vi "Plotmatrix Format Page.vi"() -> ()   [LabVIEW 2020, in "XY Plot Matrix.lvclass"]
uses:
  <vilib>/Math Plots/2D Math Plots/XY Plot Matrix/XY Plot Matrix/XY Plot Matrix.lvclass
  <vilib>/Math Plots/2D Math Plots/2D Plot/Action String/XYPlotMatrix Ctrl Act Queue.ctl
  <vilib>/Math Plots/2D Math Plots/2D Plot/Action String/XYPlotMatrix Ctrl Act Cluster.ctl
  <vilib>/Math Plots/2D Math Plots/2D Plot/Action String/2DMathPlot State Class.ctl
  <vilib>/Math Plots/2D Math Plots/2D Plot/2D Plot/Typedef/Dialog State.ctl
  <vilib>/Math Plots/2D Math Plots/2D Plot/2D Plot/Typedef/Temp Graph State.ctl
  <vilib>/Math Plots/2D Math Plots/2D Plot/2D Plot/Typedef/Temp Graph Property Action.ctl
  <vilib>/Math Plots/2D Math Plots/2D Plot/2D Plot/2D Plot.lvclass
panel:
  in  "Axis":string[](array[string])=["(X-Axis)", "(Y-Axis)"]
  in  "Current Scale":u16(ring)
  in  "Control Ref Queue":T1
  out "Format String Out":string[](array[string])
  in  "Format String In":string[](array[string])
  out "Advanced Tab":enum32{"Standard", "Advanced"}(tab)
  in  "Type":i32(listbox)
  out "Time/Date Tab":enum32{"numeric", "time"}(tab) caption="Tab Control 3"
  in  "HLP_just/pad":i32(ring) items=["Pad with spaces on left", "Pad with spaces on right", "Pad with zeros on left"]
  in  "HLP_Minimum field width":i32 caption="Minimum field width" min=0
  in  "Digits":i32 min=0
  in  "Precision Type":u16(ring) items=["Digits of precision", "Significant digits"]
  in  "HLP_exponent":bool caption="Exponent in multiples of 3"
  in  "HLP_trailing zeros":bool caption="Hide trailing zeros"
  in  "HLP_UseMinWidth":bool caption="Use minimum field width"
  in  "HLP_Date Type":u16(ring)=1 caption="Date Type" items=["Custom date format", "System date format", "Date unused"]
  in  "HLP_MDY 2-new":T2(radio)
  in  "HLP_year-new":T2(radio)
  in  "HLP_Time Type":u16(ring)=1 caption="Time Type" items=["Custom time format", "System time format", "Time unused"]
  in  "HLP_Digits":i32 caption="Digits" min=0
  in  "HLP_Hour Type-new":enum32{"Radio Selection 1", "Radio Selection 2"}(radio)
  in  "HLP_HMS-new":enum32{"Radio Selection 1", "Radio Selection 2"}(radio)
  in  "HLP_Format Code List Type":u16(ring) items=["Numeric format codes", "Relative time format codes", "Absolute time format codes"]
  in  "ODF_Format String":string caption="Format string"
  in  "HLP_percent codes":i32(listbox) caption="Numeric Format Codes"
  in  "HLP_insert format code":bool caption="Insert into Format String"
  out "HLP_Valid Fmt String":bool=TRUE caption="Valid"
  in  "HLP_Revert":bool caption="Revert"
  in  "HLP_AdvancedFmt2":enum32{"Default mode", "Advanced mode"}(radio)
  in  "Event Registration":refnum<event-registration>
  in  "Item Names":string[][][](array[string])=[[["Floating point notation", "%f"], ["Scientific notation", "%e"], ["Engineering notation", "%^e"], ["Automatic notation", "%#_g"], ["SI notation", "%p"], ["Decimal", "%d"], ["Unsigned decimal", "%u"], ["Hexadecimal", "%x"], ["Octal", "%o"], ["Binary", "%b"], ["A single percent character", "%%"], ["", ""], ["", ""], ["", ""], ["", ""], ["", ""], ["", ""], ["", ""], ["", ""], ["", ""], ["", ""], ["", ""], ["", ""]], [["Absolute time container", "%< >T"], ["Abbreviated weekday name", "%a"], ["Weekday name", "%A"], ["Abbreviated month name", "%b"], ["Month name", "%B"], ["Default date and time", "%c"], ["Day of month (01-31)", "%d"], ["Hour (24-hour clock) (00-23)", "%H"], ["Hour (12-hour clock) (01-12)", "%I"], ["Day of year (001-366)", "%j"], ["Month number (01-12)", "%m"], ["Minute (00-59)", "%M"], ["AM or PM flag", "%p"], ["Seconds (00-59)", "%S"], ["Fractional seconds with <digit>\nprecision", "%<digit> u"], ["Week number (00-53) with\nSunday as the first day of week 1", "%U"], ["Weekday number (0-6)", "%w"], ["Week number (00-53) with\nMonday as the first day of week 1", "%W"], ["Locale date", "%x"], ["Locale time", "%X"], ["Year within century (00-99)", "%y"], ["Year including century", "%Y"], ["Time zone", "%Z"]], [["Relative time container", "%< >t"], ["Weeks", "%W"], ["Days", "%D"], ["Hours", "%H"], ["Minutes", "%M"], ["Seconds", "%S"], ["Fractional seconds with <digit>\nprecision", "%<digit>u"], ["A single percent character", "%%"], ["", ""], ["", ""], ["", ""], ["", ""], ["", ""], ["", ""], ["", ""], ["", ""], ["", ""], ["", ""], ["", ""], ["", ""], ["", ""], ["", ""], ["", ""]]]
  in  "Caption Texts":string[](array[string])=["Numeric Format Codes", "Absolute Time Format Codes\n(must be within %< >T)", "Relative Time Format Codes\n(must be within %< >t)"]
  out "Format test string":string
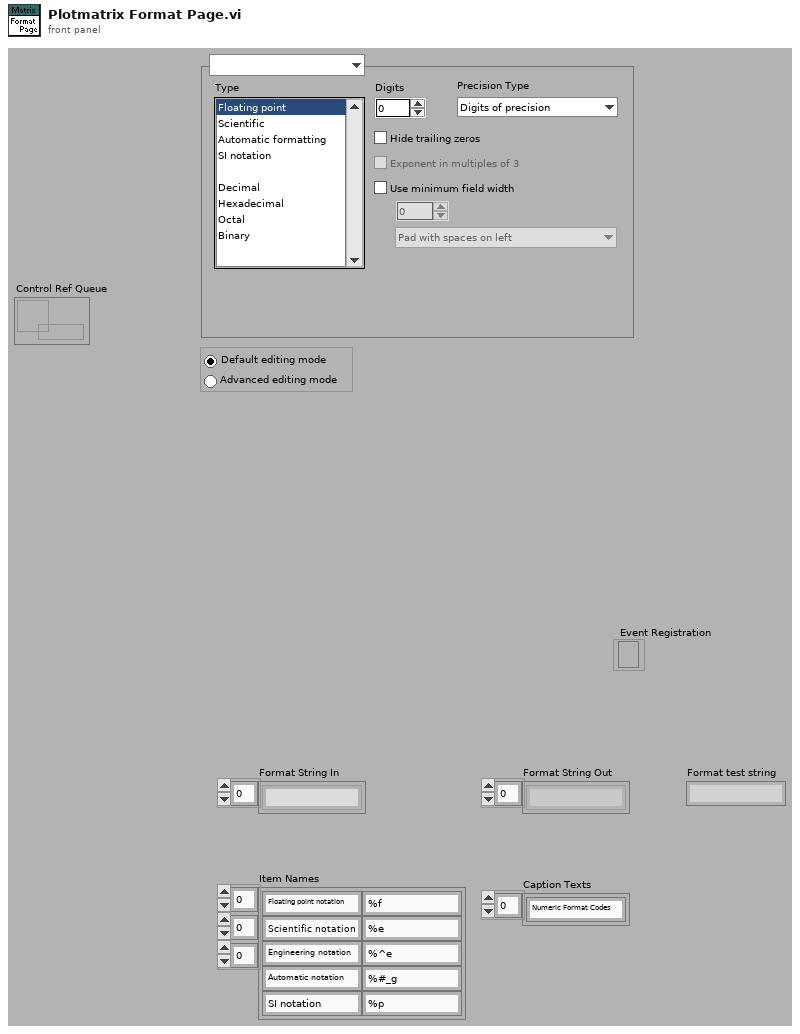
[diagram p1: front panel]
types:
  T1 = typedef "XYPlotMatrix Ctrl Act Queue.ctl" = refnum<queue>
  T2 = enum32{"Radio Selection 1", "Radio Selection 2", "Radio Selection 3"}
  T3 = typedef "2D Plot.lvclass/Dialog State.ctl" = enum16{"Initialize", "Read Property", "Write Property", "Idle", "Exit"}
  T4 = typedef "2D Plot.lvclass/Temp Graph State.ctl" = enum16{"Create", "Update Graph", "Update Property Only", "Get Plot Name", "Get Axis Name", "Destory"}
  T5 = typedef "2D Plot.lvclass/Temp Graph Property Action.ctl" = enum16{"Appearance Property", "Format Property", "Plots Property", "Scales Property"}
  T6 = enum16{"number", "absolute time", "relative time"}
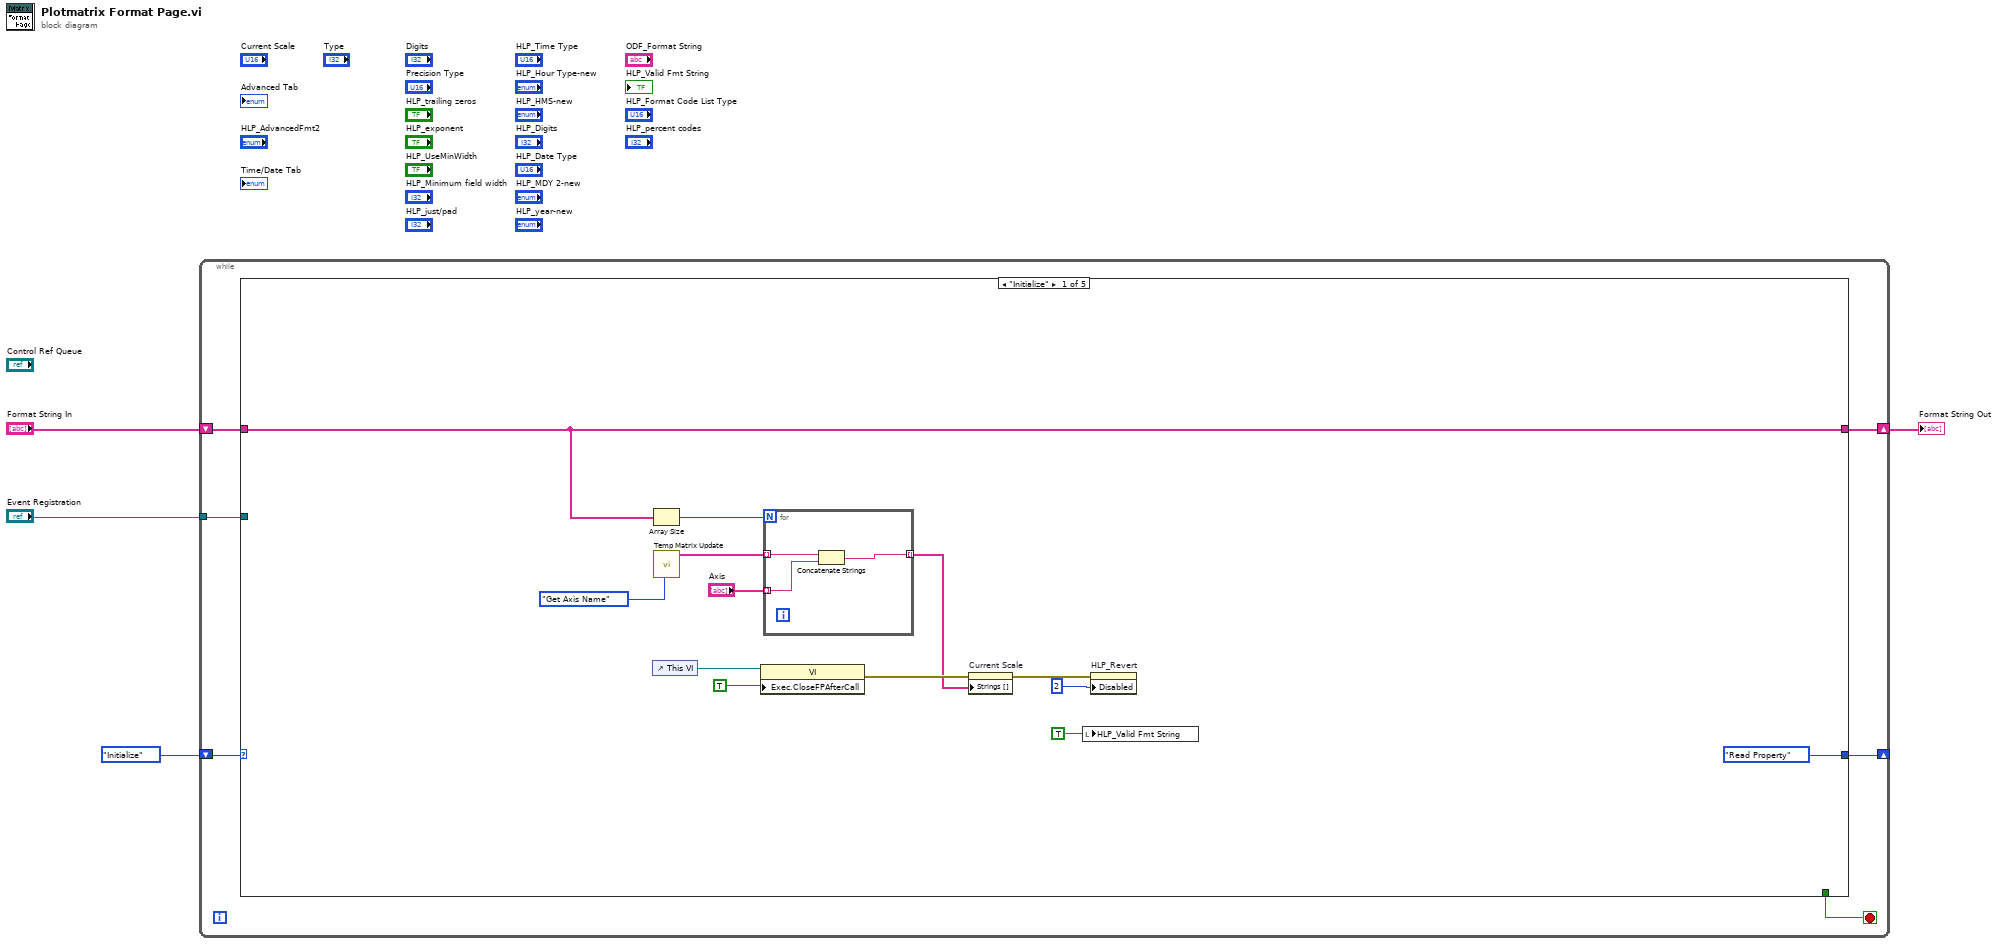
[diagram p0: block diagram]
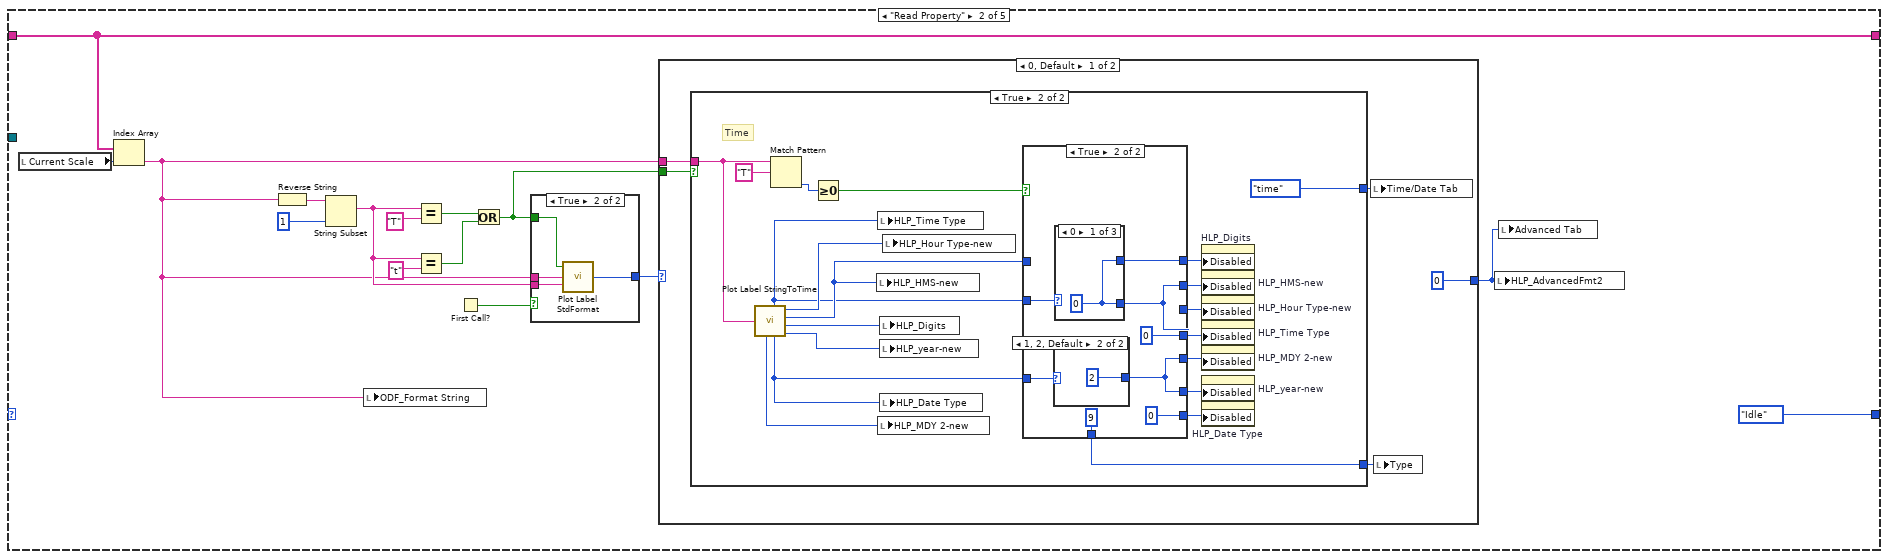
[diagram p2: hidden frame]
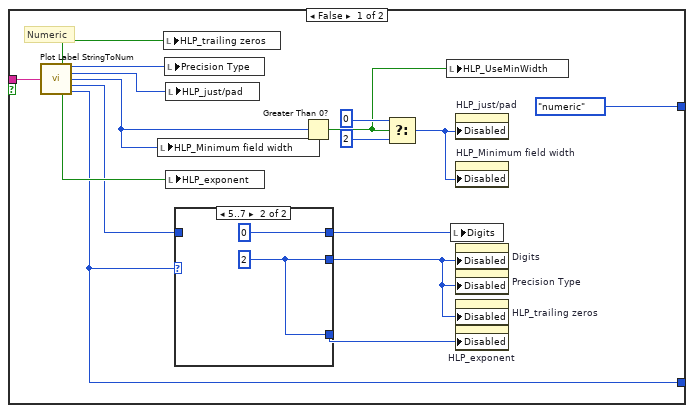
[diagram p3: hidden frame]
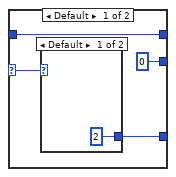
[diagram p4: hidden frame]
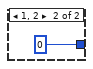
[diagram p5: hidden frame]
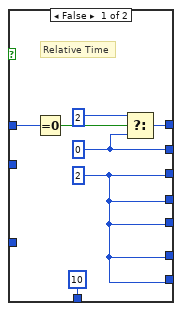
[diagram p6: hidden frame]
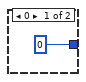
[diagram p7: hidden frame]
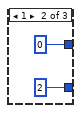
[diagram p8: hidden frame]
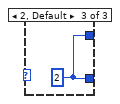
[diagram p9: hidden frame]
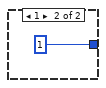
[diagram p10: hidden frame]
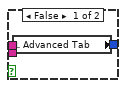
[diagram p11: hidden frame]
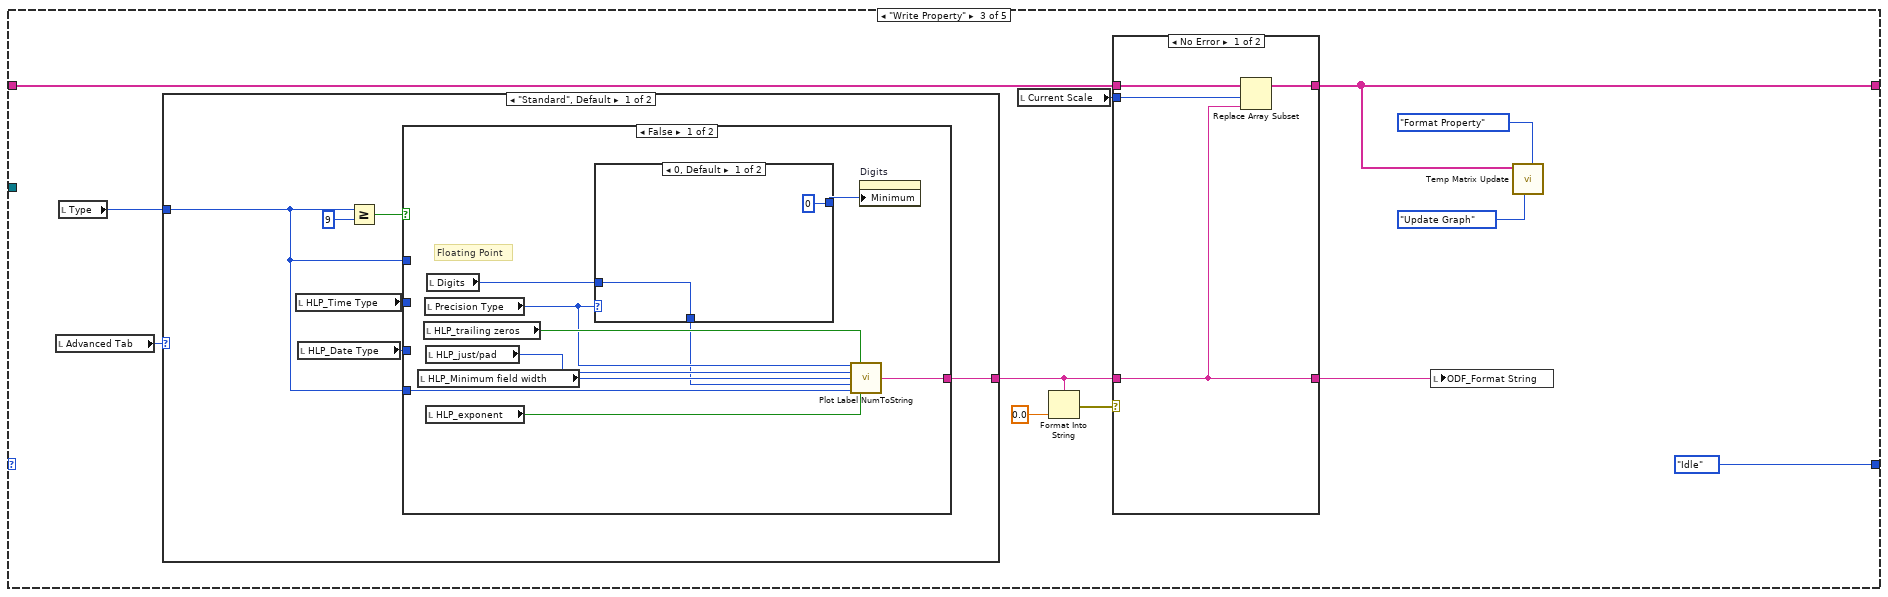
[diagram p12: hidden frame]
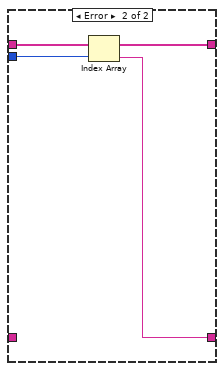
[diagram p13: hidden frame]
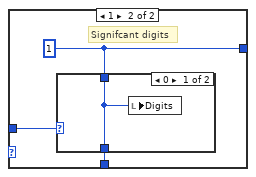
[diagram p14: hidden frame]
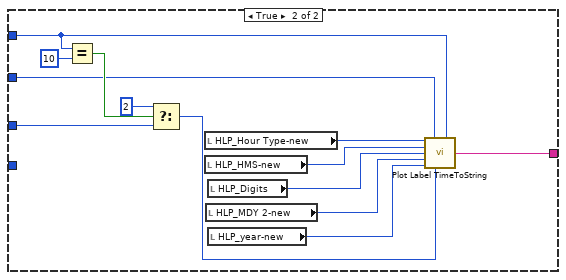
[diagram p16: hidden frame]
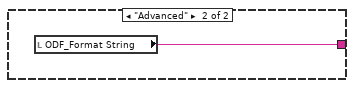
[diagram p17: hidden frame]
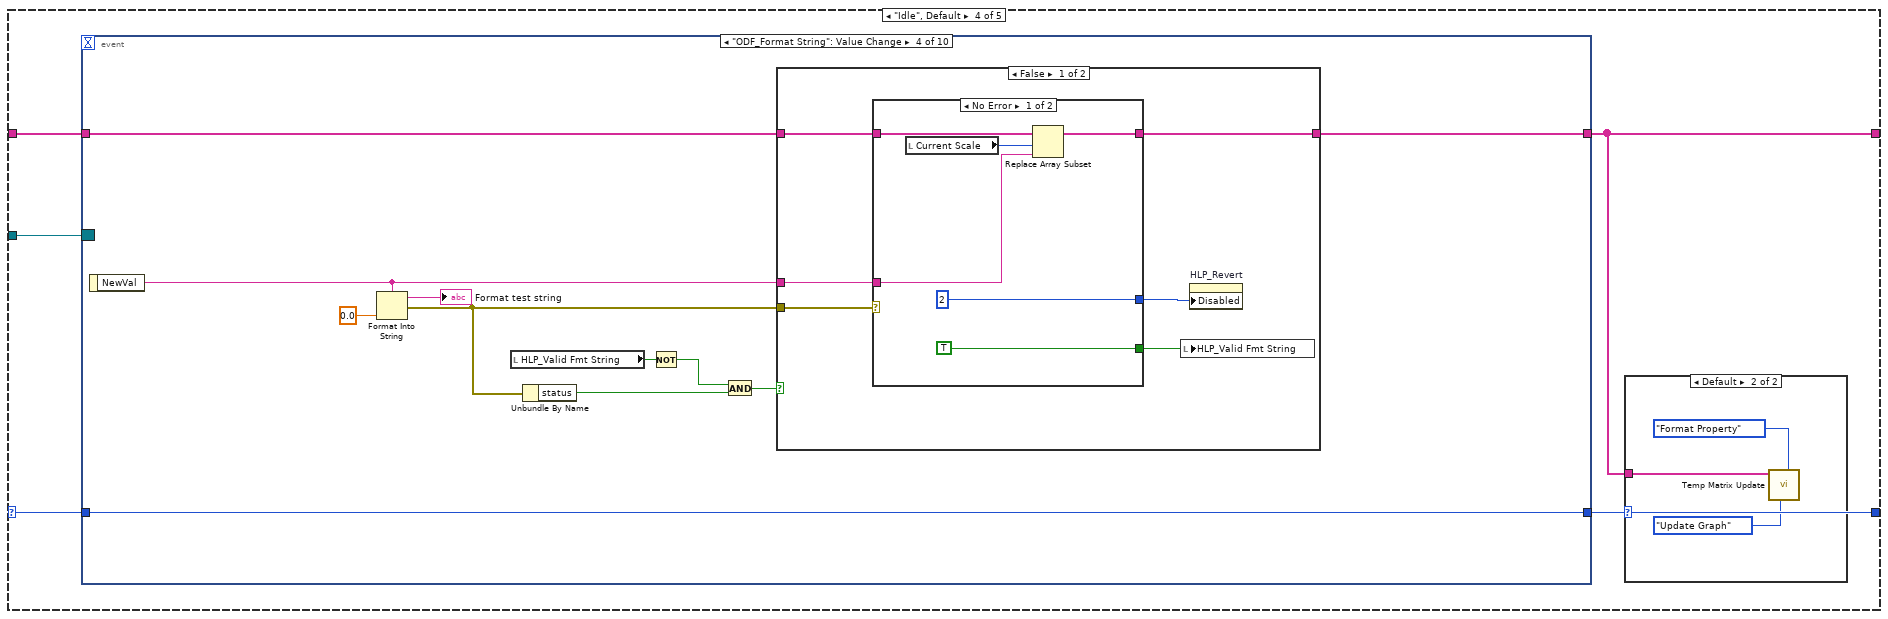
[diagram p18: hidden frame]
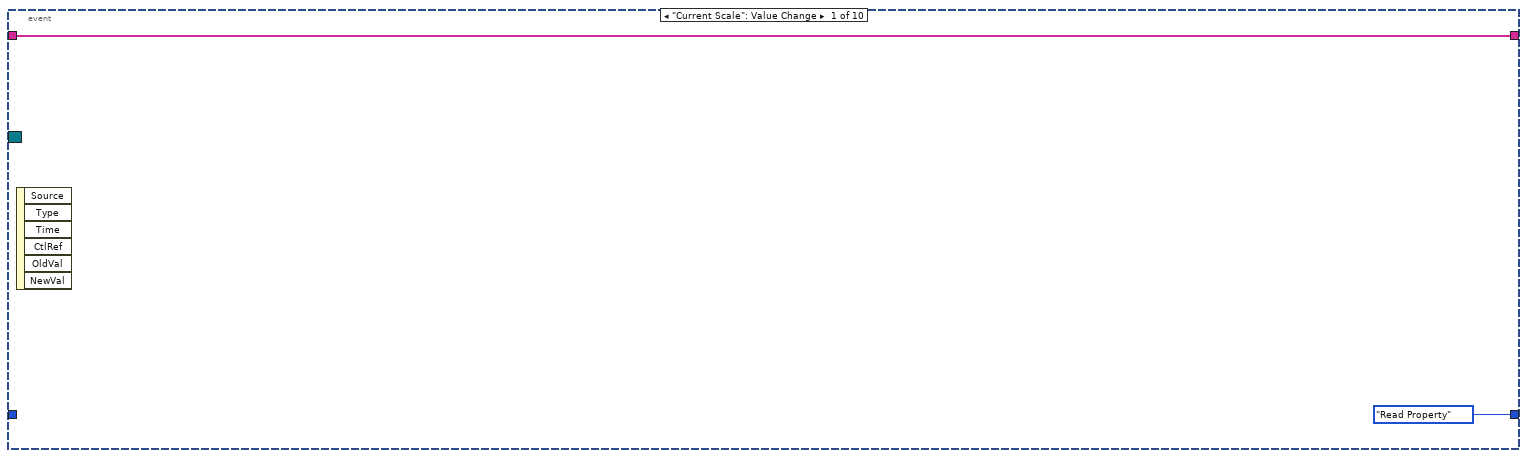
[diagram p20: hidden frame]
diagram:
  n1 = while {
    shift-right: [w5] -> w2
    shift-left: "Format String In" -> [w10]
    shift-right: [w6] -> _
    shift-left: Dialog_State."Initialize" ("Enum") -> [w7]
    tunnel: "Event Registration" -> [w8]
    stop <- w9 stop-if-true
    n2 = case shown="\"Initialize\"" w7 {
      selector: w7 -> [_ _ _ w176 _]
      tunnel: w10 -> [w13 w40 w121 w178 w401]
      tunnel: [w13 w40 w118 w175 w401] -> w5
      tunnel: [Dialog_State."Read Property" ("Enum") Dialog_State."Idle" ("Enum") Dialog_State."Idle" ("Enum") w174 Dialog_State."Exit" ("Enum")] -> w6
      tunnel: [_ _ _ _ TRUE] -> w9
      tunnel: w8 -> [_ _ _ w177 _]
      frame "Initialize" {
        n3 = control-ref of="This VI"() -> (w23:refnum<vi>)
        n4 = Array Size(array=w13) -> (size(s)=w12:i32)
        n5 = call <vilib>:"Temp Matrix Update.vi"("State"=Temp_Graph_State."Get Axis Name") -> ("Item Strings"=w15:string[])  [unwired: 4 in, 6 out]
        n6 = property class="VI"(reference=w23, "Exec.CloseFPAfterCall"=TRUE ("Execution:Close After Call")) -> (error out=w18:errorcluster)  [unwired: 1 in, 1 out]
        n7 = for {
          N: w12 -> [_]
          tunnel: w15 -> [w26] mode=indexing
          tunnel: [w24] -> w14 mode=indexing
          tunnel: "Axis" -> [w25] mode=indexing
          n8 = Concatenate Strings(w26, w25) -> (w24:string)
        }
        n9 = property on="Current Scale" class="Ring (strict)"(error in=w18, "Strings []"=w14) -> (error out=w17:errorcluster)  [unwired: 1 in, 1 out]
        n10 = local write "HLP_Valid Fmt String"(TRUE ("HLP_Valid Fmt String")) -> ()
        n11 = property on="HLP_Revert" class="Bool"(error in=w17, "Disabled"=u8 2) -> ()  [unwired: 1 in, 2 out]
      }
      frame "Read Property" {
        n12 = local read "Current Scale"() -> (w41:u16)
        n13 = Index Array(array=w40, index=w41) -> (element=w30:string)
        n14 = Reverse String(1:w30) -> (0:w35:string)
        n15 = String Subset(string=w35, length (rest)=1 ("length (rest)")) -> (substring=w39:string)  [unwired: 1 out]
        n16 = local write "ODF_Format String"(w30) -> ()
        n17 = Equal?(x=w39, y="T") -> (x = y?=w37:bool)
        n18 = Equal?(x=w39, y="t") -> (x = y?=w38:bool)
        n19 = First Call?() -> (First Call?: T/F=w32:bool)
        n20 = Or(x=w37, y=w38) -> (x .or. y?=w29:bool)
        n21 = case shown="True" w32 {
          tunnel: w39 -> [_ w115]
          tunnel: w29 -> [_ w117]
          tunnel: w30 -> [_ w116]
          tunnel: [w113 w114] -> w31
          frame False {
            n22 = local read "Advanced Tab"() -> (w113:enum32{"Standard", "Advanced"})
          }
          frame True {
            n23 = call <vilib>:"Plot Label StdFormat.vi"("Time Type"=w115, "Format String"=w116, "Type (false = numeric)"=w117) -> ("Custom"=w114:i32)
          }
        }
        n24 = case shown="0, Default" w31 {
          tunnel: w30 -> [w46 _]
          tunnel: w29 -> [w45 _]
          tunnel: [0 1] -> w28
          frame 0, Default {
            n25 = case shown="True" w45 {
              tunnel: w46 -> [w62 w88]
              tunnel: [w55 w79] -> w44
              tunnel: [enum32{"numeric", "time"}."numeric" ("Time/Date Tab") enum32{"numeric", "time"}."time" ("Time/Date Tab")] -> w43
              frame False {
                # "Numeric"
                n26 = call <vilib>:"Plot Label StringToNum.vi"("Format String"=w62) -> ("Hide trailing zeros"=w61:bool, "Digit Type"=w59:i32, "just/pad"=w58:i32, "Minimum Field Width"=w50:i32, "Digits of Precision"=w57:i32, "exponent"=w60:bool, "Numeric Format"=w55:i32)  [unwired: 8 out]
                n27 = local write "HLP_Minimum field width"(w50) -> ()
                n28 = local write "HLP_trailing zeros"(w61) -> ()
                n29 = local write "Precision Type"(w59) -> ()
                n30 = local write "HLP_just/pad"(w58) -> ()
                n31 = local write "HLP_exponent"(w60) -> ()
                n32 = case shown="5..7" w55 {
                  selector: w55 -> [w64 _]
                  tunnel: [u8 0 w69] -> w54
                  tunnel: w57 -> [w65 _]
                  tunnel: [w65 0 ("Digits of Precision")] -> w56
                  tunnel: [w63 w69] -> w53
                  frame Default {
                    n33 = case shown="Default" w64 {
                      tunnel: [u8 2 u8 0] -> w63
                      frame Default {
                      }
                      frame 1, 2 {
                      }
                    }
                  }
                  frame 5..7 {
                    w69 = u8 2
                  }
                }
                n34 = Greater Than 0?(x=w50) -> (x > 0?=w49:bool)
                n35 = Select(t=u8 0, s=w49, f=u8 2) -> (s? t:f=w48:u8)
                n36 = local write "HLP_UseMinWidth"(w49) -> ()
                n37 = local write "Digits"(w56) -> ()
                n38 = property on="HLP_just/pad" class="Ring (strict)"("Disabled"=w48) -> ()  [unwired: 2 in, 2 out]
                n39 = property on="HLP_Minimum field width" class="DigNum (strict)"("Disabled"=w48) -> ()  [unwired: 2 in, 2 out]
                n40 = property on="Digits" class="DigNum (strict)"("Disabled"=w54) -> ()  [unwired: 2 in, 2 out]
                n41 = property on="Precision Type" class="Ring (strict)"("Disabled"=w54) -> ()  [unwired: 2 in, 2 out]
                n42 = property on="HLP_trailing zeros" class="Bool (strict)"("Disabled"=w54) -> ()  [unwired: 2 in, 2 out]
                n43 = property on="HLP_exponent" class="Bool (strict)"("Disabled"=w53) -> ()  [unwired: 2 in, 2 out]
              }
              frame True {
                # "Time"
                n44 = call <vilib>:"Plot Label StringToTime.vi"("Time & Date Format String"=w88) -> ("MDY"=w86:i16, "Time Format"=w82:i16, "AM/PM"=w87:i16, "included seconds"=w83:i16, "Date Format"=w81:i16, "seconds precision"=w84:i16, "Year Format"=w85:i16)  [unwired: 3 out]
                n45 = Match Pattern(string=w88, regular expression="T") -> (offset past match=w90:i32)  [unwired: 4 out]
                n46 = Greater Or Equal To 0?(x=w90) -> (x >= 0?=w80:bool)
                n47 = local write "HLP_HMS-new"(w83) -> ()
                n48 = local write "HLP_Time Type"(w82) -> ()
                n49 = local write "HLP_MDY 2-new"(w86) -> ()
                n50 = local write "HLP_Digits"(w84) -> ()
                n51 = local write "HLP_year-new"(w85) -> ()
                n52 = local write "HLP_Date Type"(w81) -> ()
                n53 = local write "HLP_Hour Type-new"(w87) -> ()
                n54 = case shown="True" w80 {
                  tunnel: [w92 w105] -> w76
                  tunnel: [w97 w105] -> w75
                  tunnel: [w91 w98] -> w77
                  tunnel: [w97 0] -> w74
                  tunnel: [w97 0] -> w71
                  tunnel: [w97 w102] -> w72
                  tunnel: [w97 w102] -> w73
                  tunnel: w82 -> [_ w101]
                  tunnel: w81 -> [_ w100]
                  tunnel: [10 9] -> w79
                  tunnel: w83 -> [w93 _]
                  frame False {
                    w92 = 0
                    w97 = 2
                    # "Relative Time"
                    n55 = Equal To 0?(x=w93) -> (x = 0?=w94:bool)
                    n56 = Select(t=2, s=w94, f=w92) -> (s? t:f=w91:i32)
                  }
                  frame True {
                    n57 = case shown="1, 2, Default" w100 {
                      tunnel: [0 2] -> w102
                      frame 0 {
                      }
                      frame 1, 2, Default {
                      }
                    }
                    n58 = case shown="0" w101 {
                      tunnel: [w108 2 w111] -> w105
                      tunnel: [w108 0 w111] -> w98
                      frame 0 {
                        w108 = 0
                      }
                      frame 1 {
                      }
                      frame 2, Default {
                        w111 = 2
                      }
                    }
                  }
                }
                n59 = property on="HLP_Digits" class="DigNum (strict)"("Disabled"=w77) -> ()  [unwired: 2 in, 2 out]
                n60 = property on="HLP_HMS-new" class="RadioBtnsControl (strict)"("Disabled"=w76) -> ()  [unwired: 2 in, 2 out]
                n61 = property on="HLP_Hour Type-new" class="RadioBtnsControl (strict)"("Disabled"=w75) -> ()  [unwired: 2 in, 2 out]
                n62 = property on="HLP_Time Type" class="Ring (strict)"("Disabled"=w74) -> ()  [unwired: 2 in, 2 out]
                n63 = property on="HLP_MDY 2-new" class="RadioBtnsControl (strict)"("Disabled"=w73) -> ()  [unwired: 2 in, 2 out]
                n64 = property on="HLP_year-new" class="RadioBtnsControl (strict)"("Disabled"=w72) -> ()  [unwired: 2 in, 2 out]
                n65 = property on="HLP_Date Type" class="Ring (strict)"("Disabled"=w71) -> ()  [unwired: 2 in, 2 out]
              }
            }
            n66 = local write "Time/Date Tab"(w43) -> ()
            n67 = local write "Type"(w44) -> ()
          }
          frame 1 {
          }
        }
        n68 = local write "HLP_AdvancedFmt2"(w28) -> ()
        n69 = local write "Advanced Tab"(w28) -> ()
      }
      frame "Write Property" {
        n70 = local read "Advanced Tab"() -> (w129:enum32{"Standard", "Advanced"})
        n71 = local read "Type"() -> (w128:i32)
        n72 = case shown="\"Standard\", Default" w129 {
          tunnel: w128 -> [w140 _]
          tunnel: [w137 w173] -> w125
          frame "Standard", Default {
            n73 = local read "HLP_Time Type"() -> (w139:u16)
            n74 = local read "HLP_Date Type"() -> (w138:u16)
            n75 = Greater Or Equal?(x=w140, y=9) -> (x >= y?=w141:bool)
            n76 = case shown="False" w141 {
              tunnel: w140 -> [_ w167]
              tunnel: w140 -> [w151 _]
              tunnel: w139 -> [_ w168]
              tunnel: w138 -> [_ w169]
              tunnel: [w152 w160] -> w137
              frame False {
                # "Floating Point"
                n77 = local read "HLP_Minimum field width"() -> (w149:i32)
                n78 = local read "HLP_trailing zeros"() -> (w148:bool)
                n79 = local read "Precision Type"() -> (w146:u16)
                n80 = local read "HLP_just/pad"() -> (w147:i32)
                n81 = local read "HLP_exponent"() -> (w150:bool)
                n82 = local read "Digits"() -> (w145:i32)
                n83 = case shown="0, Default" w146 {
                  tunnel: w145 -> [w153 w157]
                  tunnel: [0 ("Data Range:Minimum") w156] -> w144
                  tunnel: [w153 w155] -> w143
                  frame 0, Default {
                  }
                  frame 1 {
                    w156 = 1 ("Data Range:Minimum")
                    # "Signifcant digits"
                    n84 = case shown="0" w157 {
                      selector: w157 -> [_ w159]
                      tunnel: w156 -> [w158 _]
                      tunnel: [w158 w159] -> w155
                      frame 0 {
                        n85 = local write "Digits"(w158) -> ()
                      }
                      frame 1, Default {
                      }
                    }
                  }
                }
                n86 = call <vilib>:"Plot Label NumToString.vi"("Digit Type"=w146, "Hide trailing zeros"=w148, "just/pad"=w147, "Minimum Field Width"=w149, "Digits of Precision"=w143, "Numeric Format"=w151, "exponent"=w150) -> ("Format String"=w152:string)  [unwired: 8 out]
                n87 = property on="Digits" class="DigNum (strict)"("Minimum"=w144) -> ()  [unwired: 2 in, 2 out]
              }
              frame True {
                n88 = Equal?(x=w167, y=10) -> (x = y?=w170:bool)
                n89 = Select(t=u16 2, s=w170, f=w169) -> (s? t:f=w161:u16)
                n90 = local read "HLP_Hour Type-new"() -> (w166:enum32{"Radio Selection 1", "Radio Selection 2"})
                n91 = local read "HLP_HMS-new"() -> (w165:enum32{"Radio Selection 1", "Radio Selection 2"})
                n92 = local read "HLP_MDY 2-new"() -> (w163:T2)
                n93 = local read "HLP_Digits"() -> (w164:i32)
                n94 = local read "HLP_year-new"() -> (w162:T2)
                n95 = call <vilib>:"Plot Label TimeToString.vi"("AM/PM"=w166, "Time Format"=w168, "Type (10 = Absolute)"=w167, "included seconds"=w165, "seconds precision"=w164, "m-d-y sequence"=w163, "year format"=w162, "Date Format"=w161) -> ("Format String"=w160:string)  [unwired: 3 in, 4 out]
              }
            }
          }
          frame "Advanced" {
            n96 = local read "ODF_Format String"() -> (w173:string)
          }
        }
        n97 = local read "Current Scale"() -> (w124:u16)
        n98 = Format Into String(format string=w125, 0.0 ("input 1")) -> (error out=w126:errorcluster)  [unwired: 2 in, 1 out]
        n99 = case shown="No Error" w126 {
          tunnel: w121 -> [w133 w134]
          tunnel: [w132 w134] -> w118
          tunnel: w125 -> [w130 _]
          tunnel: w124 -> [w131 w136]
          tunnel: [w130 w135] -> w123
          frame No Error {
            n100 = Replace Array Subset(array=w133, new element=w130, index=w131) -> (w132:string[])
          }
          frame Error {
            n101 = Index Array(array=w134, index=w136) -> (element=w135:string)
          }
        }
        n102 = local write "ODF_Format String"(w123) -> ()
        n103 = call <vilib>:"Temp Matrix Update.vi"("Property Name"=Temp_Graph_Property_Action."Format Property", "State"=Temp_Graph_State."Update Graph", "Property In"=w118) -> ()  [unwired: 2 in, 7 out]
      }
      frame "Idle", Default {
        n104 = event shown="[3] \"ODF_Format String\": Value Change" {
          selector: w177 -> [_ _ _ _ _ _ _ _ _ _]
          dyn-events: _ -> [_ _ _ _ _ _ _ _ _ _]
          timeout: _ -> [_ _ _ _ _ _ _ _ _ _]
          tunnel: w178 -> [w183 w185 w189 w260 w288 w294 w304 w372 w379 w399]
          tunnel: [w183 w185 w189 w259 w288 w294 w304 w372 w379 w399] -> w175
          tunnel: [Dialog_State."Read Property" ("Enum") Dialog_State."Write Property" ("Enum") Dialog_State."Write Property" ("Enum") w267 w289 Dialog_State."Write Property" ("Enum") w300 w371 w378 Dialog_State."Exit" ("Enum")] -> w174
          tunnel: w176 -> [_ _ _ w267 w289 _ w299 w371 w378 _]
          event "Current Scale": Value Change {
            n105 = event-data() -> ()  [unwired: 7 out]
          }
          event "HLP_Digits", "Digits", "HLP_just/pad", "HLP_exponent", "HLP_trailing zeros", "Precision Type", "HLP_Hour Type-new", "HLP_MDY 2-new", "HLP_year-new": Value Change {
            n106 = event-data() -> ()  [unwired: 7 out]
          }
          event "HLP_Date Type", "HLP_Time Type", "Type", "HLP_Minimum field width", "HLP_HMS-new": Value Change {
            n107 = event-data() -> ()  [unwired: 7 out]
            n108 = local read "HLP_AdvancedFmt2"() -> (w191:enum32{"Default mode", "Advanced mode"})
            n109 = local read "Type"() -> (w187:i32)
            n110 = case shown="Default" w187 {
              selector: w187 -> [w192 _]
              tunnel: [w192 u8 5] -> w186
              frame Default {
              }
              frame 6..8 {
              }
            }
            n111 = local write "Type"(w186) -> ()
            n112 = case shown="\"Default mode\", Default" w191 {
              tunnel: w186 -> [w201 _]
              tunnel: [u32 0 u32 1] -> w190
              frame "Default mode", Default {
                n113 = case shown="Default" w201 {
                  selector: w201 -> [w250 _]
                  tunnel: [u8 0 w255] -> w210
                  tunnel: [w251 w255] -> w211
                  frame Default {
                    n114 = case shown="1, 2" w250 {
                      tunnel: [u8 2 u8 0] -> w251
                      frame Default {
                      }
                      frame 1, 2 {
                      }
                    }
                  }
                  frame 5..8 {
                    w255 = u8 2
                  }
                }
                n115 = Greater Or Equal?(x=w201, y=9) -> (x >= y?=w213:bool)
                n116 = Equal?(x=w201, y=10) -> (x = y?=w202:bool)
                n117 = Boolean To (0,1)(Boolean=w213) -> (0, 1=w212:i16)
                n118 = local write "Time/Date Tab"(w212) -> ()
                n119 = property on="HLP_exponent" class="Bool (strict)"("Disabled"=w211) -> ()  [unwired: 2 in, 2 out]
                n120 = property on="Precision Type" class="Ring (strict)"("Disabled"=w210) -> ()  [unwired: 2 in, 2 out]
                n121 = property on="HLP_trailing zeros" class="Bool (strict)"("Disabled"=w210) -> ()  [unwired: 2 in, 2 out]
                n122 = property on="Digits" class="DigNum (strict)"("Disabled"=w210) -> ()  [unwired: 2 in, 2 out]
                n123 = local read "HLP_Minimum field width"() -> (w207:i32)
                n124 = case shown="False" w202 {
                  tunnel: [w220 w246] -> w200
                  tunnel: [w219 w245] -> w199
                  tunnel: [w215 w244] -> w198
                  tunnel: [w218 w244] -> w197
                  tunnel: [w217 w244] -> w196
                  tunnel: [w216 w244] -> w195
                  tunnel: [w215 w244] -> w194
                  frame False {
                    w215 = u8 0
                    n125 = local read "HLP_Time Type"() -> (w222:u16)
                    n126 = local read "HLP_Date Type"() -> (w221:u16)
                    n127 = call <vilib>:"Plot subChangeDetector.vi"("value"=w222) -> ("changed?"=w223:bool)  [unwired: 10 out]
                    n128 = Equal?(x=2, y=w222) -> (x = y?=w226:bool)
                    n129 = Equal?(x=2, y=w221) -> (x = y?=w225:bool)
                    n130 = And(x=w226, y=w225) -> (x .and. y?=w224:bool)
                    n131 = case shown="False" w224 {
                      tunnel: w223 -> [_ w241]
                      tunnel: w222 -> [w233 _]
                      tunnel: w221 -> [w232 _]
                      tunnel: [w231 w240] -> w220
                      tunnel: [w230 w240] -> w219
                      tunnel: [w230 w240] -> w218
                      tunnel: [w229 w240] -> w217
                      tunnel: [w229 w240] -> w216
                      frame False {
                        n132 = case shown="1" w233 {
                          tunnel: [w236 u8 2 w239] -> w230
                          tunnel: [w236 u8 0 w239] -> w231
                          frame 0 {
                            w236 = u8 0
                          }
                          frame 1 {
                          }
                          frame 2, Default {
                            w239 = u8 2
                          }
                        }
                        n133 = case shown="0" w232 {
                          tunnel: [u8 0 u8 2] -> w229
                          frame 0 {
                          }
                          frame 1, 2, Default {
                          }
                        }
                      }
                      frame True {
                        w240 = u8 2
                        n134 = case shown="False" w241 {
                          frame False {
                            w242 = u16 1 items=["Custom Date Format", "System Date Format", "Date Unused"] ("Date Type")
                            n135 = local write "HLP_Date Type"(w242) -> ()
                          }
                          frame True {
                            w243 = u16 1 items=["Custom Time Format", "System Time Format", "Time Unused"] ("Time Type")
                            n136 = local write "HLP_Time Type"(w243) -> ()
                          }
                        }
                      }
                    }
                  }
                  frame True {
                    w244 = u8 2
                    w245 = u8 0
                    # "Relative Time"
                    n137 = local read "HLP_HMS-new"() -> (w247:enum32{"Radio Selection 1", "Radio Selection 2"})
                    n138 = Equal To 0?(x=w247) -> (x = 0?=w249:bool)
                    n139 = Select(t=u8 2, s=w249, f=w245) -> (s? t:f=w246:u8)
                  }
                }
                n140 = Greater Than 0?(x=w207) -> (x > 0?=w206:bool)
                n141 = Select(t=u8 0, s=w206, f=u8 2) -> (s? t:f=w205:u8)
                n142 = local write "HLP_UseMinWidth"(w206) -> ()
                n143 = property on="HLP_Minimum field width" class="DigNum (strict)"("Disabled"=w205) -> ()  [unwired: 2 in, 2 out]
                n144 = property on="HLP_just/pad" class="Ring (strict)"("Disabled"=w205) -> ()  [unwired: 2 in, 2 out]
                n145 = property on="HLP_Digits" class="DigNum (strict)"("Disabled"=w200) -> ()  [unwired: 2 in, 2 out]
                n146 = property on="HLP_HMS-new" class="RadioBtnsControl (strict)"("Disabled"=w199) -> ()  [unwired: 2 in, 2 out]
                n147 = property on="HLP_Hour Type-new" class="RadioBtnsControl (strict)"("Disabled"=w197) -> ()  [unwired: 2 in, 2 out]
                n148 = property on="HLP_Time Type" class="Ring (strict)"("Disabled"=w198) -> ()  [unwired: 2 in, 2 out]
                n149 = property on="HLP_MDY 2-new" class="RadioBtnsControl (strict)"("Disabled"=w196) -> ()  [unwired: 2 in, 2 out]
                n150 = property on="HLP_year-new" class="RadioBtnsControl (strict)"("Disabled"=w195) -> ()  [unwired: 2 in, 2 out]
                n151 = property on="HLP_Date Type" class="Ring (strict)"("Disabled"=w194) -> ()  [unwired: 2 in, 2 out]
              }
              frame "Advanced mode" {
              }
            }
            n152 = local write "Advanced Tab"(w190) -> ()
          }
          event "ODF_Format String": Value Change {
            n153 = event-data() -> ("NewVal"=w258:string)  [unwired: 1 out]
            n154 = Format Into String(format string=w258, 0.0 ("input 1")) -> (resulting string=→"Format test string":string, error out=w261:errorcluster)  [unwired: 2 in]
            n155 = local read "HLP_Valid Fmt String"() -> (w264:bool)
            n156 = Unbundle By Name(w261) -> ("status"=w263:bool)
            n157 = Not(x=w264) -> (.not. x?=w265:bool)
            n158 = And(x=w265, y=w263) -> (x .and. y?=w262:bool)
            n159 = case shown="False" w262 {
              tunnel: w261 -> [w273 _]
              tunnel: w260 -> [w270 w283]
              tunnel: [w269 w283] -> w259
              tunnel: w258 -> [w268 _]
              frame False {
                n160 = case shown="No Error" w273 {
                  tunnel: [TRUE FALSE] -> w272
                  tunnel: [u8 2 u8 0] -> w271
                  tunnel: w270 -> [w277 w280]
                  tunnel: [w276 w280] -> w269
                  tunnel: w268 -> [w275 _]
                  frame No Error {
                    n161 = local read "Current Scale"() -> (w274:u16)
                    n162 = Replace Array Subset(array=w277, new element=w275, index=w274) -> (w276:string[])
                  }
                  frame Error {
                  }
                }
                n163 = local write "HLP_Valid Fmt String"(w272) -> ()
                n164 = property on="HLP_Revert" class="Bool"("Disabled"=w271) -> ()  [unwired: 2 in, 2 out]
              }
              frame True {
              }
            }
          }
          event "HLP_Revert": Value Change {
            n165 = event-data() -> ()  [unwired: 7 out]
            n166 = local read "Current Scale"() -> (w287:u16)
            n167 = Index Array(array=w288, index=w287) -> (element=w286:string)
            n168 = local write "HLP_Valid Fmt String"(TRUE ("HLP_Valid Fmt String")) -> ()
            n169 = local write "ODF_Format String"(w286) -> ()
            n170 = property on="HLP_Revert" class="Bool"("Disabled"=u8 2) -> ()  [unwired: 2 in, 2 out]
          }
          event "HLP_UseMinWidth": Value Change {
            n171 = event-data() -> ("NewVal"=w293:bool)  [unwired: 1 out]
            n172 = case shown="False" w293 {
              tunnel: [u8 2 u8 0] -> w292
              tunnel: [0 1] -> w291
              frame False {
              }
              frame True {
              }
            }
            n173 = local write "HLP_Minimum field width"(w291) -> ()
            n174 = property on="HLP_just/pad" class="Ring (strict)"("Disabled"=w292) -> ()  [unwired: 2 in, 2 out]
            n175 = property on="HLP_Minimum field width" class="DigNum (strict)"("Disabled"=w292) -> ()  [unwired: 2 in, 2 out]
          }
          event "HLP_AdvancedFmt2": Value Change {
            # "Reset these booleans Reset when changing to either tab because when going to advanced, you can't have a bad format string.  When going to simple mode, we reset these because we coerce to a good format string."
            n176 = event-data() -> ("NewVal"=w305:enum32{"Default mode", "Advanced mode"})  [unwired: 1 out]
            n177 = case shown="\"Default mode\", Default" w305 {
              tunnel: w304 -> [w323 _]
              tunnel: [0 1] -> w303
              tunnel: [TRUE ("HLP_Valid Fmt String") TRUE ("HLP_Valid Fmt String")] -> w301
              tunnel: [Dialog_State."Read Property" ("Enum") w359] -> w300
              tunnel: w299 -> [_ w359]
              frame "Default mode", Default {
                # "Switching from simple to advanced editing mode.\nThis case determines if the current format string can be represented by the basic selection controls.  If not, the format string is coerced to something that can be represented by the simple controls.  When coerced, the format string property is written, to update the control.  Whether coerced or not, the next event is Read Properties so that the controls are set up properly in the UI.\n\nIf the current format string in advanced was good, we use it.  If not, we use the last known good format string.  So, switching back to simple mode is a way for users to get out of a bad format string situation."
                n178 = local read "Current Scale"() -> (w322:u16)
                n179 = local read "HLP_Valid Fmt String"() -> (w321:bool)
                n180 = local read "ODF_Format String"() -> (w309:string)
                n181 = Index Array(array=w323, index=w322) -> (element=w320:string)
                n182 = Select(t=w309, s=w321, f=w320) -> (s? t:f=w312:string)
                n183 = Reverse String(1:w312) -> (0:w319:string)
                n184 = String Subset(string=w319, length (rest)=1 ("length (rest)")) -> (substring=w311:string)  [unwired: 1 out]
                n185 = Equal?(x=w311, y="T") -> (x = y?=w316:bool)
                n186 = Equal?(x=w311, y="t") -> (x = y?=w317:bool)
                n187 = Or(x=w316, y=w317) -> (x .or. y?=w313:bool)
                n188 = case shown="False" w313 {
                  tunnel: w312 -> [w324 w356]
                  tunnel: w311 -> [_ w355]
                  tunnel: [w325 w353] -> w310
                  frame False {
                    n189 = call <vilib>:"Plot Label StdFormat.vi"("Format String"=w324) -> ("Custom"=w326:i32)  [unwired: 2 in]
                    n190 = case shown="1" w326 {
                      tunnel: [w327 w328] -> w325
                      tunnel: w324 -> [w327 w336]
                      frame 0, Default {
                        # "Not a custom value.  Keep\nformat"
                      }
                      frame 1 {
                        # "Custom format.  Coerce.\nNote, ideally the page should not\ncoerce unless the user changes format\nin the default page."
                        n191 = call <vilib>:"Plot Label StringToNum.vi"("Format String"=w336) -> ("Hide trailing zeros"=w329:bool, "Digit Type"=w334:i32, "just/pad"=w333:i32, "Minimum Field Width"=w332:i32, "Digits of Precision"=w331:i32, "exponent"=w330:bool, "Numeric Format"=w335:i32)  [unwired: 8 out]
                        n192 = case shown="Default" w335 {
                          tunnel: w335 -> [_ w345]
                          tunnel: w334 -> [_ w344]
                          tunnel: w333 -> [_ w343]
                          tunnel: w332 -> [_ w342]
                          tunnel: w331 -> [_ w341]
                          tunnel: w330 -> [_ w340]
                          tunnel: w329 -> [_ w339]
                          tunnel: ["%.0f" w338] -> w328
                          frame -1 {
                          }
                          frame Default {
                            n193 = call <vilib>:"Plot Label NumToString.vi"("Digit Type"=w344, "Hide trailing zeros"=w339, "just/pad"=w343, "Minimum Field Width"=w342, "Digits of Precision"=w341, "Numeric Format"=w345, "exponent"=w340) -> ("Format String"=w338:string)  [unwired: 8 out]
                          }
                        }
                      }
                    }
                  }
                  frame True {
                    n194 = call <vilib>:"Plot Label StringToTime.vi"("Time & Date Format String"=w356) -> ("MDY"=w347:i16, "Time Format"=w352:i16, "AM/PM"=w351:i16, "included seconds"=w350:i16, "Date Format"=w346:i16, "seconds precision"=w349:i16, "Year Format"=w348:i16)  [unwired: 3 out]
                    n195 = case shown="\"t\"" w355 {
                      tunnel: [9 10] -> w354
                      frame "T", Default {
                      }
                      frame "t" {
                      }
                    }
                    n196 = call <vilib>:"Plot Label TimeToString.vi"("AM/PM"=w351, "Time Format"=w352, "Type (10 = Absolute)"=w354, "included seconds"=w350, "seconds precision"=w349, "m-d-y sequence"=w347, "year format"=w348, "Date Format"=w346) -> ("Format String"=w353:string)  [unwired: 3 in, 4 out]
                  }
                }
                n197 = local write "ODF_Format String"(w310) -> ()
              }
              frame "Advanced mode" {
                # "Switching from advanced to simple editing mode.\nThis case sets up the correct advanced format string table based on format type.  \n\nDon't go to read or write properties because the advanced tab shows the format string and it should be kept up-to-date by other events."
                n198 = local read "Type"() -> (w367:i32)
                n199 = case shown="9" w367 {
                  tunnel: [T6."number" ("Enum") T6."absolute time" ("Enum") T6."relative time" ("Enum")] -> w366
                  frame 0, Default {
                  }
                  frame 9 {
                  }
                  frame 10 {
                  }
                }
                n200 = Index Array(array="Item Names", index (dim 0)=w366) -> (element=w362:string[][])  [unwired: 2 in]
                n201 = Index Array(array="Caption Texts", index=w366) -> (element=w363:string)
                n202 = property on="HLP_percent codes" class="MCListbox (strict)"("ItemNames"=w362, "Caption.Text"=w363) -> ()  [unwired: 2 in, 2 out]
              }
            }
            n203 = local write "HLP_Valid Fmt String"(w301) -> ()
            n204 = local write "Advanced Tab"(w303) -> ()
            n205 = property on="HLP_Revert" class="Bool"("Disabled"=u8 2) -> ()  [unwired: 2 in, 2 out]
          }
          event "HLP_Format Code List Type": Value Change {
            n206 = event-data() -> ("NewVal"=w373:u16)  [unwired: 1 out]
            n207 = local read "Item Names"() -> (w375:string[][][])
            n208 = local read "Caption Texts"() -> (w374:string[])
            n209 = Index Array(array=w375, index (dim 0)=w373) -> (element=w376:string[][])  [unwired: 2 in]
            n210 = Index Array(array=w374, index=w373) -> (element=w377:string)
            n211 = property on="HLP_percent codes" class="MCListbox (strict)"("ItemNames"=w376, "Caption.Text"=w377) -> ()  [unwired: 2 in, 2 out]
          }
          event "HLP_insert format code": Value Change; "HLP_percent codes": Double Click {
            n212 = event-data() -> ()  [unwired: 5 out]
            n213 = property on="HLP_percent codes" class="MCListbox (strict)"() -> (error out=w380:errorcluster, "ItemNames"=w395:string[][], "Value"=w393:i32)  [unwired: 2 in, 1 out]
            n214 = local read "ODF_Format String"() -> (w387:string)
            n215 = property on="ODF_Format String" class="Str"(error in=w380) -> (error out=w382:errorcluster, "Text.Selection Start"=w385:u32)  [unwired: 1 in, 1 out]
            n216 = Index Array(array=w395, index (row)=w393, index (col)=1 ("disabled index (col)")) -> (element=w384:string)
            n217 = String Length(string=w384) -> (length=w392:i32)
            n218 = Add(x=w392, y=w385) -> (x+y=w391:u32)
            n219 = Search/Split String(string=w387, offset (0)=w385) -> (substring before match=w389:string, match + rest of string=w388:string)  [unwired: 2 out]
            n220 = property on="ODF_Format String" class="Str"(error in=w382, "Text.Selection Start"=w391, "Text.Selection End"=w391, "Key Focus"=TRUE) -> (error out=w381:errorcluster)  [unwired: 1 in, 1 out]
            n221 = Concatenate Strings(w389, w384, w388) -> (w386:string)
            n222 = case shown="\"No Error\", Default" w386 {
              selector: w386 -> [_ w397]
              tunnel: w387 -> [w396 _]
              tunnel: [w396 w397] -> w383
              frame "Error" {
              }
              frame "No Error", Default {
              }
            }
            n223 = property on="ODF_Format String" class="Str"(error in=w381, "Val(Sgnl)"=w383) -> ()  [unwired: 1 in, 2 out]
          }
          event User Event {
            n224 = event-data() -> ()  [unwired: 6 out]
          }
        }
        n225 = case shown="Default" w174 {
          tunnel: w175 -> [_ w180]
          frame "Write Property", "Exit" {
          }
          frame Default {
            n226 = call <vilib>:"Temp Matrix Update.vi"("Property Name"=Temp_Graph_Property_Action."Format Property", "State"=Temp_Graph_State."Update Graph", "Property In"=w180) -> ()  [unwired: 2 in, 7 out]
          }
        }
      }
      frame "Exit" {
      }
    }
  }
  "Format String Out" <- w2
